vi "33500B Ramp_init.vi"(0 "Waveform":T1(ring), 1 "Frquency":dbl=66.76 format="%#_13g", 2 "Burst ON/off":bool=TRUE, 3 "Power ON/off":bool=TRUE, 4 "Symmetry":dbl=13.0 format="%#_13g", 5 "Phase":dbl=-24.0 format="%#_13g", 6 "Amp(vpp)":dbl=1.0 format="%#_13g", 7 "offset with pace interval(s)":dbl=0.06 format="%#_13g", 8 "Pace Rate":string="60", 9 "VISA资源名称":refnum<visa-resource-name>="TCPIP0::192.168.40.72:INSTR") -> (14 "VISA资源名称输出":refnum<visa-resource-name>)   [LabVIEW 2016]
panel:
  out "读取缓冲区":string
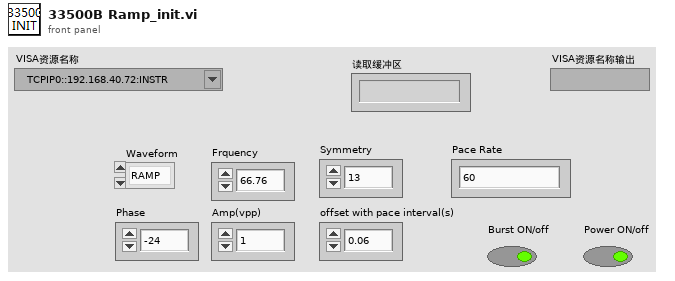
[diagram p1: front panel]
types:
  T1 = enum16{"RAMP", "SINusoid", "SQUare", "TRIangle", "PULSe", "PRBS", "ARB", "DC", "NOISe"}
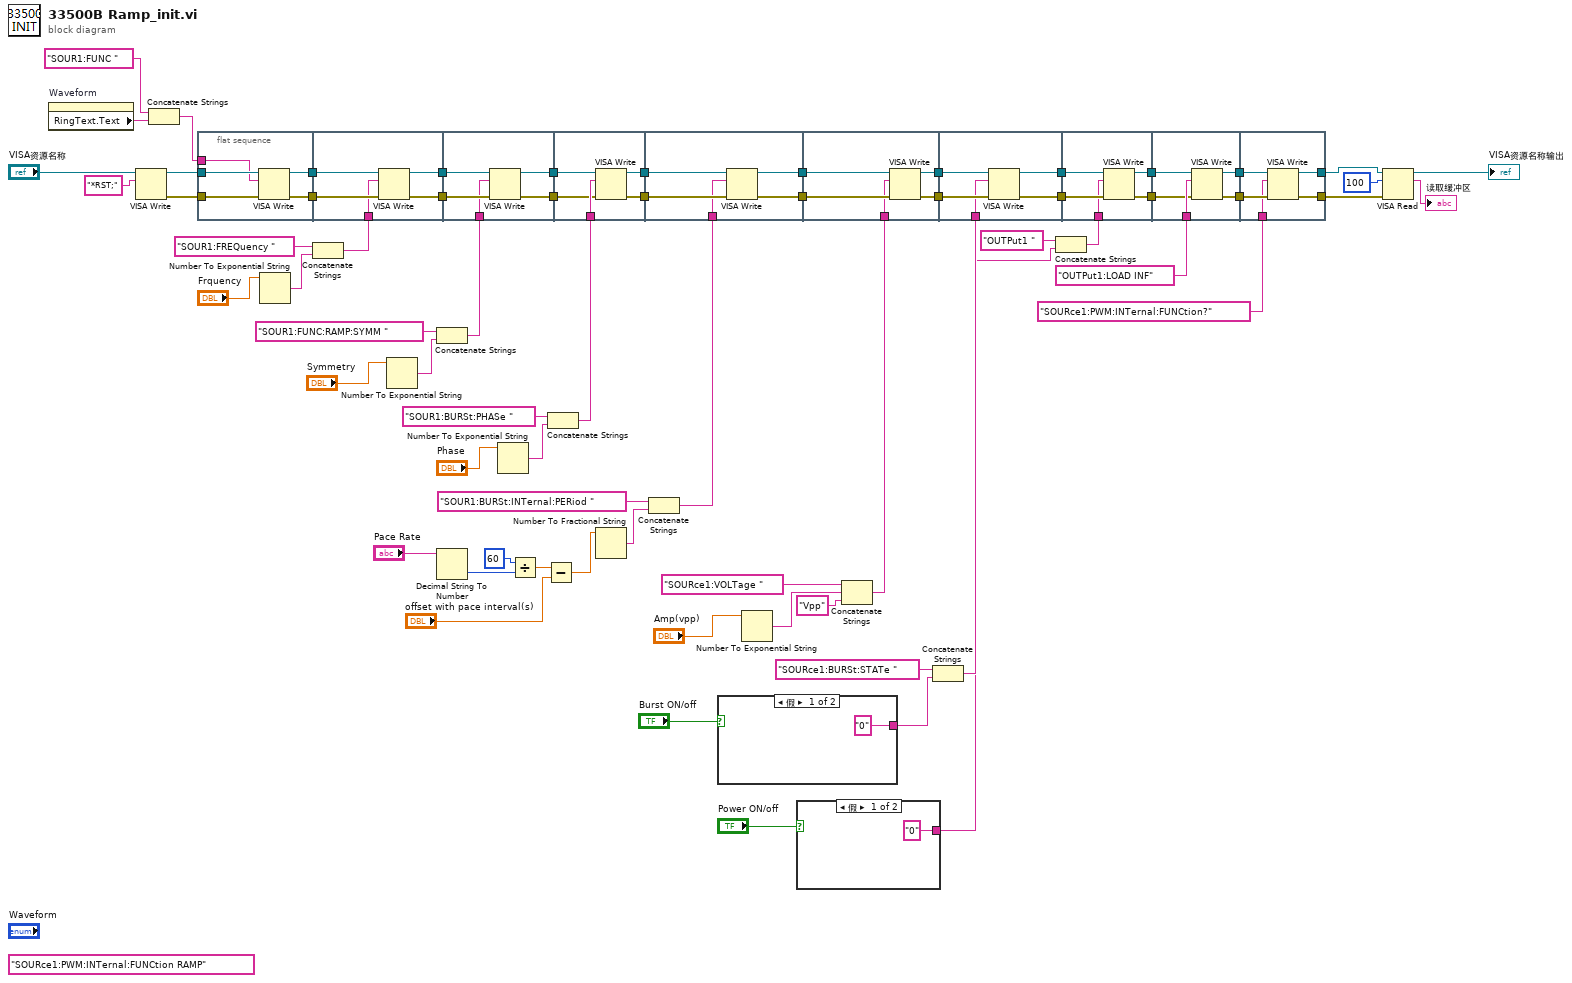
[diagram p0: block diagram]
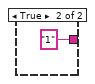
[diagram p2: hidden frame]
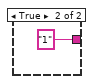
[diagram p3: hidden frame]
diagram:
  (unwired) "SOURce1:PWM:INTernal:FUNCtion RAMP" ("写入缓冲区")
  n1 = property on="Waveform" class="Enum (严格)"() -> ("RingText.Text"=w36:string)  [unwired: 2 in, 2 out]
  n2 = VISA Write(VISA resource name="VISA资源名称", write buffer="*RST;" ("写入缓冲区")) -> (VISA resource name out=w64:refnum<visa-resource-name>, error out=w59:errorcluster)  [unwired: 1 in, 1 out]
  n3 = Concatenate Strings("SOUR1:FUNC " ("写入缓冲区"), w36) -> (w35:string)
  n4 = flat-sequence {
    tunnel: w59 -> [w70]
    tunnel: w64 -> [w71]
    tunnel: [w69] -> w56
    tunnel: [w68] -> w55
    tunnel: w35 -> [w67]
    tunnel: w56 -> [w76]
    tunnel: [w73] -> w54
    tunnel: w55 -> [w75]
    tunnel: [w74] -> w53
    tunnel: w31 -> [w72]
    tunnel: w54 -> [w81]
    tunnel: [w80] -> w52
    tunnel: w53 -> [w79]
    tunnel: [w78] -> w51
    tunnel: w27 -> [w77]
    tunnel: w52 -> [w86]
    tunnel: w51 -> [w83]
    tunnel: [w82] -> w50
    tunnel: [w85] -> w48
    tunnel: w23 -> [w84]
    tunnel: w50 -> [w89]
    tunnel: [w87] -> w49
    tunnel: w48 -> [w91]
    tunnel: [w90] -> w47
    tunnel: w38 -> [w88]
    tunnel: [w96] -> w58
    tunnel: [w95] -> w57
    tunnel: w49 -> [w93]
    tunnel: w47 -> [w94]
    tunnel: w18 -> [w92]
    tunnel: w58 -> [w98]
    tunnel: w57 -> [w101]
    tunnel: [w100] -> w12
    tunnel: [w99] -> w11
    tunnel: w15 -> [w97]
    tunnel: w12 -> [w106]
    tunnel: [w104] -> w5
    tunnel: w11 -> [w105]
    tunnel: [w103] -> w3
    tunnel: w7 -> [w102]
    tunnel: w5 -> [w110]
    tunnel: [w108] -> w4
    tunnel: w3 -> [w109]
    tunnel: [w107] -> w2
    tunnel: "OUTPut1:LOAD INF" ("写入缓冲区") -> [w111]
    tunnel: [w113] -> w62
    tunnel: [w114] -> w63
    tunnel: w4 -> [w115]
    tunnel: w2 -> [w116]
    tunnel: "SOURce1:PWM:INTernal:FUNCtion?" ("写入缓冲区") -> [w112]
    frame #0 {
      n5 = VISA Write(VISA resource name=w71, write buffer=w67, error in (no error)=w70) -> (VISA resource name out=w69:refnum<visa-resource-name>, error out=w68:errorcluster)  [unwired: 1 out]
    }
    frame #1 {
      n6 = VISA Write(VISA resource name=w76, write buffer=w72, error in (no error)=w75) -> (VISA resource name out=w73:refnum<visa-resource-name>, error out=w74:errorcluster)  [unwired: 1 out]
    }
    frame #2 {
      n7 = VISA Write(VISA resource name=w81, write buffer=w77, error in (no error)=w79) -> (VISA resource name out=w80:refnum<visa-resource-name>, error out=w78:errorcluster)  [unwired: 1 out]
    }
    frame #3 {
      n8 = VISA Write(VISA resource name=w86, write buffer=w84, error in (no error)=w83) -> (VISA resource name out=w85:refnum<visa-resource-name>, error out=w82:errorcluster)  [unwired: 1 out]
    }
    frame #4 {
      n9 = VISA Write(VISA resource name=w91, write buffer=w88, error in (no error)=w89) -> (VISA resource name out=w90:refnum<visa-resource-name>, error out=w87:errorcluster)  [unwired: 1 out]
    }
    frame #5 {
      n10 = VISA Write(VISA resource name=w94, write buffer=w92, error in (no error)=w93) -> (VISA resource name out=w95:refnum<visa-resource-name>, error out=w96:errorcluster)  [unwired: 1 out]
    }
    frame #6 {
      n11 = VISA Write(VISA resource name=w101, write buffer=w97, error in (no error)=w98) -> (VISA resource name out=w100:refnum<visa-resource-name>, error out=w99:errorcluster)  [unwired: 1 out]
    }
    frame #7 {
      n12 = VISA Write(VISA resource name=w106, write buffer=w102, error in (no error)=w105) -> (VISA resource name out=w104:refnum<visa-resource-name>, error out=w103:errorcluster)  [unwired: 1 out]
    }
    frame #8 {
      n13 = VISA Write(VISA resource name=w110, write buffer=w111, error in (no error)=w109) -> (VISA resource name out=w108:refnum<visa-resource-name>, error out=w107:errorcluster)  [unwired: 1 out]
    }
    frame #9 {
      n14 = VISA Write(VISA resource name=w115, write buffer=w112, error in (no error)=w116) -> (VISA resource name out=w114:refnum<visa-resource-name>, error out=w113:errorcluster)  [unwired: 1 out]
    }
  }
  n15 = Number To Exponential String(number="Frquency") -> (E-format string=w33:string)  [unwired: 3 in]
  n16 = Concatenate Strings("SOUR1:FREQuency " ("写入缓冲区"), w33) -> (w31:string)
  n17 = Number To Exponential String(number="Symmetry") -> (E-format string=w30:string)  [unwired: 3 in]
  n18 = Concatenate Strings("SOUR1:FUNC:RAMP:SYMM " ("写入缓冲区"), w30) -> (w27:string)
  n19 = Decimal String To Number(string="Pace Rate") -> (number=w45:i32)  [unwired: 2 in, 1 out]
  n20 = Number To Exponential String(number="Phase") -> (E-format string=w25:string)  [unwired: 3 in]
  n21 = Divide(x=60, y=w45) -> (x/y=w43:dbl)
  n22 = Subtract(x=w43, y="offset with pace interval(s)") -> (x-y=w41:dbl)
  n23 = Concatenate Strings("SOUR1:BURSt:PHASe " ("写入缓冲区"), w25) -> (w23:string)
  n24 = Number To Fractional String(number=w41) -> (F-format string=w39:string)  [unwired: 3 in]
  n25 = Concatenate Strings("SOUR1:BURSt:INTernal:PERiod " ("写入缓冲区"), w39) -> (w38:string)
  n26 = case shown="假" "Burst ON/off" {
    tunnel: ["0" "1"] -> w13
    frame False {
    }
    frame True {
    }
  }
  n27 = Number To Exponential String(number="Amp(vpp)") -> (E-format string=w22:string)  [unwired: 3 in]
  n28 = case shown="假" "Power ON/off" {
    tunnel: ["0" "1"] -> w10
    frame False {
    }
    frame True {
    }
  }
  n29 = Concatenate Strings("SOURce1:VOLTage " ("写入缓冲区"), w22, "Vpp" ("字符串")) -> (w18:string)
  n30 = Concatenate Strings("SOURce1:BURSt:STATe " ("写入缓冲区"), w13) -> (w15:string)
  n31 = Concatenate Strings("OUTPut1 " ("写入缓冲区"), w10) -> (w7:string)
  n32 = VISA Read(VISA resource name=w63, byte count=u32 100 ("字节总数"), error in (no error)=w62) -> (VISA resource name out=→"VISA资源名称输出":refnum<visa-resource-name>, read buffer=→"读取缓冲区":string)  [unwired: 2 out]
